vi "dispose context.vi"(8 "error in":errorcluster, 11 "lvlibcrypto digest in":refnum<class "lvlibcrypto cipher.lvclass">) -> (0 "error out":errorcluster)   [LabVIEW 2016, in "lvlibcrypto cipher.lvclass"]
uses:
  lvlibcrypto cipher.lvclass
  lvlibcrypto cipher.lvclass/lvlibcrypto cipher.ctl
  lv tls dll.lvlib
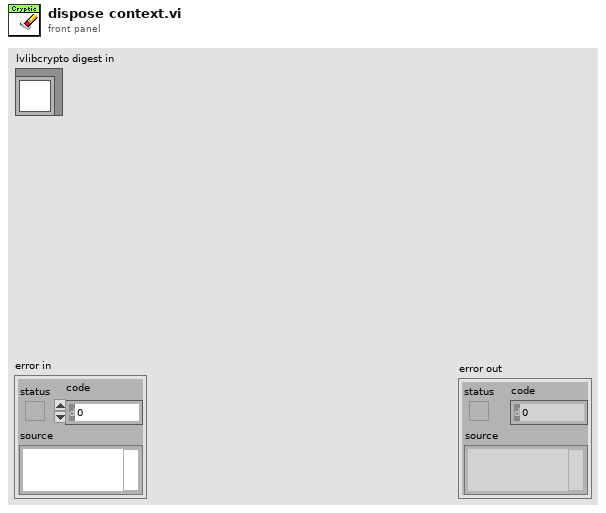
[diagram p1: front panel]
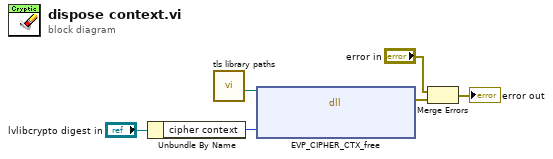
[diagram p0: block diagram]
diagram:
  n1 = Unbundle By Name("lvlibcrypto digest in") -> ("cipher context"=w4:u64)
  n2 = call "tls library paths.vi"() -> ("libcrypto"=w5:path)  [unwired: 8 in, 3 out]
  n3 = dll-call lib="C:/Users/IEUser/Desktop/tlssimple/libcrypto-41.dll" fn="EVP_CIPHER_CTX_free"(path in=w5, "context"=w4) -> (error out=w1:errorcluster)  [unwired: 4 in, 1 out]
  n4 = Merge Errors("error in", w1) -> (→"error out":errorcluster)
